vi "NetworkMultichannelSpectrometerTest.vi"() -> ()   [LabVIEW 2015]
panel:
  in  "Enter the \nInetegration Time":i32=20000
  in  "Channel Index":i32
  in  "Ip Address":string="10.120.17.67"
  out "Spectrum of the first Spectrometer":cluster{"Y":dbl[], "Y":dbl[]}[](graph)
  in  "stop":bool
  in  "Start":bool
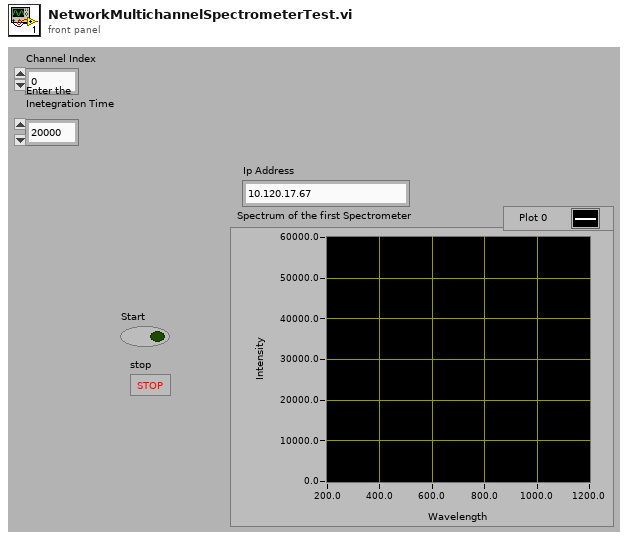
[diagram p1: front panel]
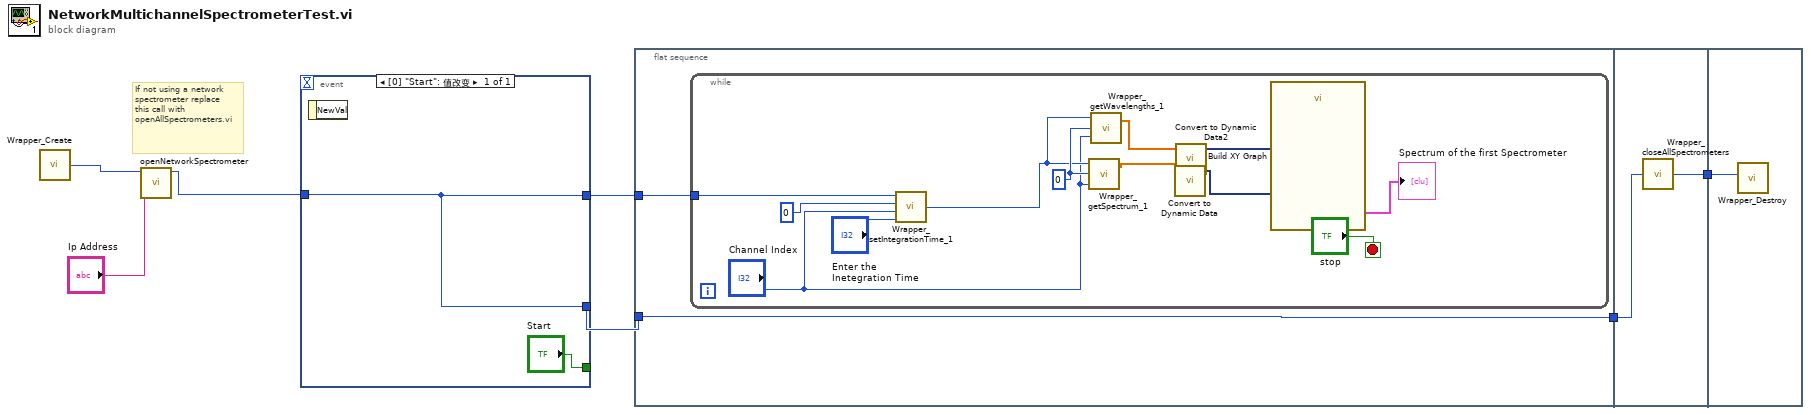
[diagram p0: block diagram]
diagram:
  # "If not using a network spectrometer replace\nthis call with openAllSpectrometers.vi"
  n1 = call "Wrapper_Create.vi"() -> ("Wrapper"=w3:u32)
  n2 = call "openNetworkSpectrometer.vi"("Ip Address"="Ip Address", "Wrapper"=w3) -> ("Wrapper"=w2:u32)  [unwired: 9 out]
  n3 = event shown="[0] \"Start\": 值改变" {
    selector: _ -> [_]
    dyn-events: _ -> [_]
    timeout: _ -> [_]
    tunnel: ["Start"] -> _
    tunnel: w2 -> [w8]
    tunnel: [w8] -> w7
    tunnel: [w8] -> w5
    event "Start": Value Change {
      n4 = event-data() -> ()  [unwired: 2 out]
    }
  }
  n5 = flat-sequence {
    tunnel: w7 -> [w11]
    tunnel: [w10] -> w6
    tunnel: w5 -> [w10]
    tunnel: w6 -> [w25]
    tunnel: [w24] -> w4
    tunnel: w4 -> [w26]
    frame #0 {
      n6 = while {
        tunnel: w11 -> [w16]
        stop <- "stop" stop-if-true
        w17 = 0 ("Index")
        n7 = call "Wrapper_setIntegrationTime_1.vi"("Integration Time"="Enter the \nInetegration Time", "Channel Index"="Channel Index", "Spectrometer Index"=0 ("Index"), "Wrapper In"=w16) -> ("Wrapper Out"=w15:u32)
        n8 = call "Wrapper_getSpectrum_1.vi"("Channel Index"="Channel Index", "Index"=w17, "Wrapper"=w15) -> ("Spectrum Values"=w19:dbl[])  [unwired: 1 out]
        n9 = call "Wrapper_getWavelengths_1.vi"("Channel Index"="Channel Index", "Index"=w17, "Wrapper"=w15) -> ("WL Values"=w18:dbl[])  [unwired: 1 out]
        n10 = call "Convert to Dynamic Data"("Array"=w19) -> ("Dynamic Data Type"=w21:dynamicdata)  [unwired: 3 out]
        n11 = call "Convert to Dynamic Data2"("Array"=w18) -> ("Dynamic Data Type"=w20:dynamicdata)  [unwired: 3 out]
        n12 = call "Build XY Graph"("Y Input"=w21, "X Input"=w20) -> ("XY Graph"=→"Spectrum of the first Spectrometer":cluster{"Y":dbl[], "Y":dbl[]}[])  [unwired: 3 in, 6 out]
      }
    }
    frame #1 {
      n13 = call "Wrapper_closeAllSpectrometers.vi"("Wrapper In"=w25) -> ("Wrapper Out"=w24:u32)
    }
    frame #2 {
      n14 = call "Wrapper_Destroy.vi"("Wrapper"=w26) -> ()
    }
  }
